vi "Misc Timeout Counter.vi"(8 "error in (no error)":errorcluster, 10 "number of tries (3)":i32=3) -> (0 "error out":errorcluster)   [LabVIEW 2011, in "Misc VIs.lvlib"]
doc: "Ignores timeout error for an specified number of times (number of tries).\nAn external counter must be provided."
uses:
  Misc VIs.lvlib
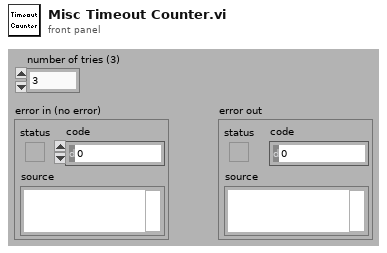
[diagram p1: front panel]
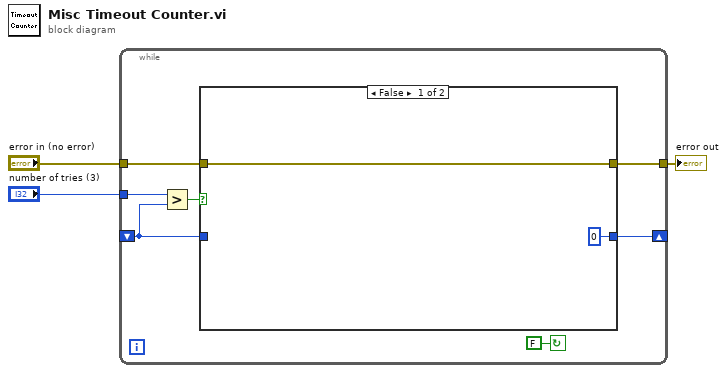
[diagram p0: block diagram]
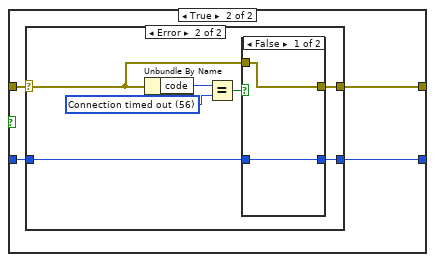
[diagram p2: hidden frame]
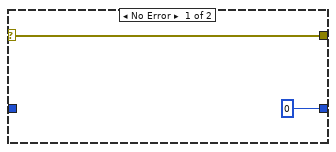
[diagram p3: hidden frame]
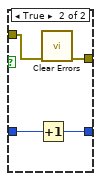
[diagram p4: hidden frame]
diagram:
  n1 = while {
    tunnel: [w9] -> w3
    tunnel: "error in (no error)" -> [w8]
    tunnel: "number of tries (3)" -> [w7]
    shift-right: [w4] -> _
    shift-left: _ -> [w6]
    stop <- FALSE continue-if-true
    n2 = Greater?(x=w7, y=w6) -> (0:w10:bool)
    n3 = case shown="False" w10 {
      tunnel: w8 -> [w12 w16]
      tunnel: [w12 w15] -> w9
      tunnel: w6 -> [_ w14]
      tunnel: [0 ("t") w13] -> w4
      frame False {
      }
      frame True {
        n4 = case shown="Error" w16 {
          selector: w16 -> [w18 w19]
          tunnel: [w18 w22] -> w15
          tunnel: w14 -> [_ w21]
          tunnel: [0 ("t") w20] -> w13
          frame No Error {
          }
          frame Error {
            w24 = 56 items=["No Error", "Argument Error", "Memory Full", "Out of Zone", "End of File", "File Already Open", "Generic File IO Error", "File Not Found", "File Permission Error", "Disk Full", "Duplicate Path", "Too Many Files Open", "Not Enabled", "Resource File Not Found", "Cannot Add Resource", "Resource Not Found", "Image Not Found", "Image Memory Error", "Pen Does Not Exist", "Config Bad Type", "Config Token Not Found", "Config Parse Error", "Config Memory Error", "Bad External Code Format", "Bad External Code Offset", "External Code Not Present", "Null Window", "Destroy Window Mixup", "Null Menu", "Print Aborted", "Bad Print Record", "Print Driver Error", "Windows Error During Print", "Memory Error During Print", "Print Dialog Error", "Generic Print Error", "Invalid Device Refnum", "Device Not Found", "Device Parameter Error", "Device Unit Error", "Can't Open Device", "Device Call Aborted", "Generic Error", "Cancelled By User", "Object ID Too Low", "Object ID Too High", "Object Not In Heap", "Unknown Heap", "Bad DefProc ID", "DefProc Not In Table", "Message Out Of Range", "Null Method", "Unknown Message", "Manager Call Not Supported", "Bad address", "Connection In progress", "Connection timed out", "Connection is already in progress", "Network attribute not supported", "Network error", "Address in use", "System out of memory", "Connection aborted", "Connection refused", "Connection is not connected", "Connection is already connected", "Connection closed", "Initialize error (interapplication manager)", "Bad occurrence", "Wait on unbound occurrence handler", "Occurrence queue overflow", "Bad path", "Semaphore not signaled", "Unrecognized type (interapplication manager)"] ("1st Error to Convert")
            n5 = Unbundle By Name(w19) -> ("code"=w25:i32)
            n6 = Equal?(x=w25, y=w24) -> (x = y?=w23:bool)
            n7 = case shown="False" w23 {
              tunnel: [w27 w31] -> w22
              tunnel: w21 -> [w26 w30]
              tunnel: [w26 w29] -> w20
              tunnel: w19 -> [w27 w28]
              frame False {
              }
              frame True {
                n8 = Increment(x=w30) -> (x+1=w29:i32)
                n9 = call <vilib>:"Clear Errors.vi"("error in (no error)"=w28) -> ("error out"=w31:errorcluster)  [unwired: 6 in]
              }
            }
          }
        }
      }
    }
  }
  "error out" <- w3
